vi "ReplaceSymbolValue.vi"(8 "error in (no error)":errorcluster, 11 "SetConditionalSymbol in":refnum<class "SetConditionalSymbol.lvclass">) -> (0 "error out":errorcluster, 1 "Output/Failure":string, 2 "Success?":bool, 3 "SetConditionalSymbol out":refnum<class "SetConditionalSymbol.lvclass">)   [LabVIEW 2020, in "SetConditionalSymbol.lvclass"]
doc: "Sets the value of the conditional disable symbol to what was provided to the LabVIEWCLI."
uses:
  SetConditionalSymbol.lvclass
  SetConditionalSymbol.lvclass/SetConditionalSymbol.ctl
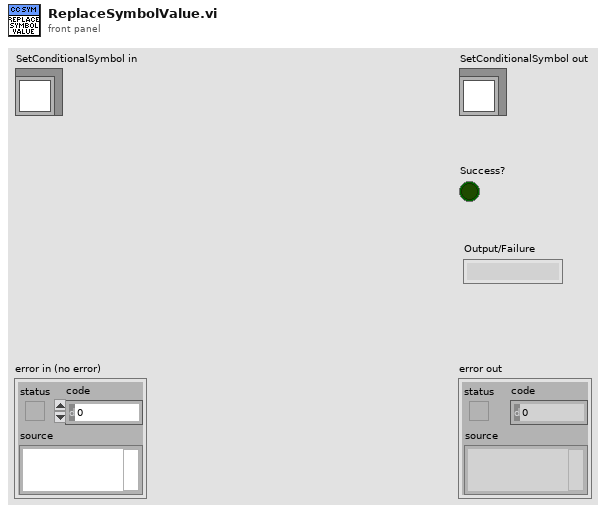
[diagram p1: front panel]
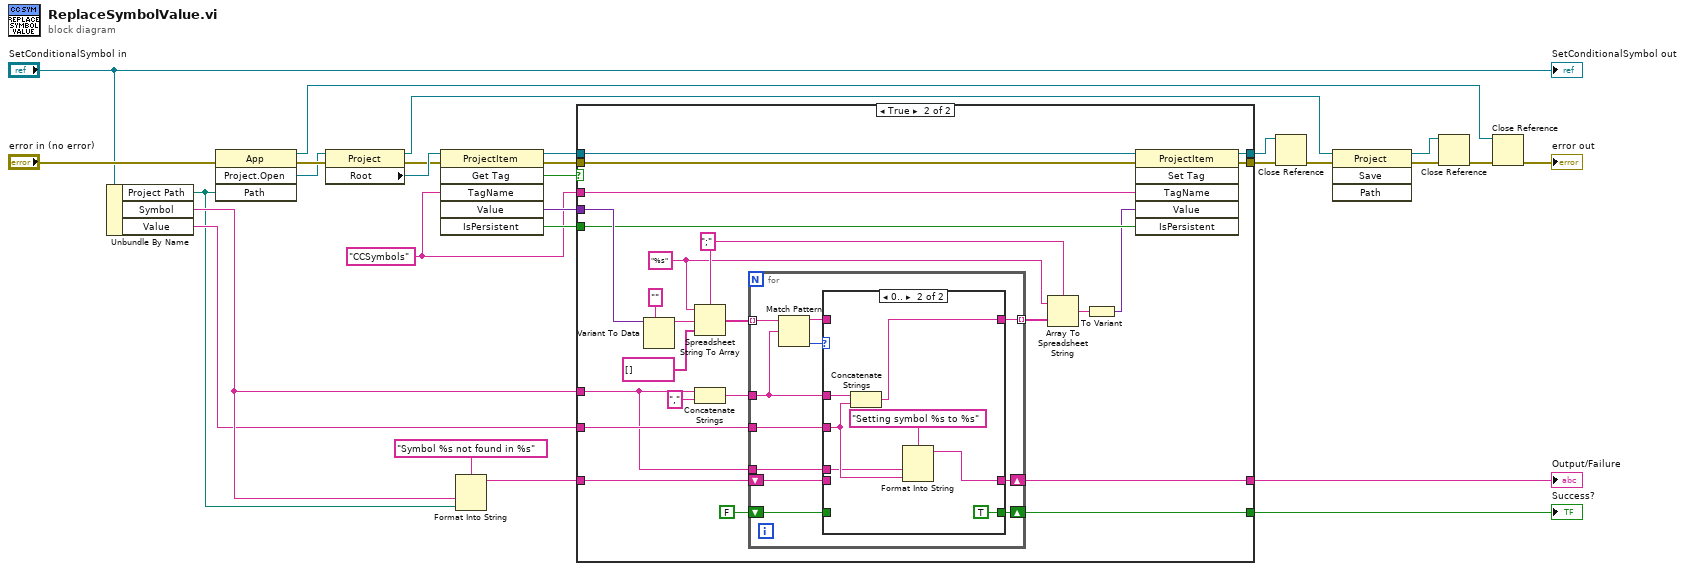
[diagram p0: block diagram]
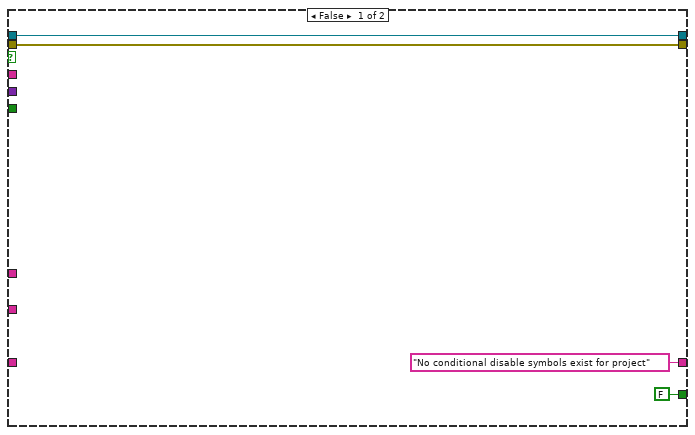
[diagram p2: hidden frame]
diagram:
  w19 = "CCSymbols" ("Tag Name")
  n1 = Unbundle By Name("SetConditionalSymbol in") -> ("Project Path"=w2:path, "Symbol"=w4:string, "Value"=w3:string)
  n2 = invoke class="App" method="Project.Open"(error in="error in (no error)", "Path"=w2) -> (reference out=w7:refnum<vi>, error out=w12:errorcluster, "Project:Open"=w11:refnum<vi>)  [unwired: 2 in, 1 out]
  n3 = property class="Project"(reference=w11, error in=w12) -> (reference out=w8:refnum<vi>, error out=w13:errorcluster, "Root"=w14:refnum<vi>)
  n4 = invoke class="ProjectItem" method="Get Tag"(reference=w14, error in=w13, "TagName"=w19) -> (reference out=w21:refnum<vi>, error out=w22:errorcluster, "GetTag"=w23:bool, "Value"=w24:variant, "IsPersistent"=w20:bool)  [unwired: 3 in, 1 out]
  n5 = Format Into String(format string="Symbol %s not found in %s" ("Tag Name"), w4, w2) -> (resulting string=w5:string)  [unwired: 2 in, 1 out]
  n6 = case shown="True" w23 {
    tunnel: w24 -> [_ w56]
    tunnel: w4 -> [_ w36]
    tunnel: w3 -> [_ w49]
    tunnel: w22 -> [w32 w44]
    tunnel: w21 -> [w31 w43]
    tunnel: [w32 w42] -> w10
    tunnel: [w31 w41] -> w9
    tunnel: w20 -> [_ w40]
    tunnel: w19 -> [_ w38]
    tunnel: w5 -> [_ w37]
    tunnel: ["No conditional disable symbols exist for project" w35] -> w25
    tunnel: [FALSE w33] -> w1
    frame False {
    }
    frame True {
      w46 = "%s" ("format string")
      w47 = ";" ("delimiter (Tab)")
      n7 = Variant To Data(type="", Variant=w56) -> (data=w54:string)  [unwired: 1 in, 1 out]
      n8 = Spreadsheet String To Array(delimiter (Tab)=w47, format string=w46, spreadsheet string=w54, array type (2D Dbl)=string[] []) -> (array=w52:string[])
      n9 = Concatenate Strings(w36, "," ("string")) -> (w50:string)
      n10 = for {
        tunnel: w52 -> [w66] mode=indexing
        tunnel: w50 -> [w62]
        tunnel: w49 -> [w63]
        tunnel: [w65] -> w48 mode=indexing
        shift-right: [w60] -> w35
        shift-left: w37 -> [w61]
        tunnel: w36 -> [w59]
        shift-right: [w57] -> w33
        shift-left: FALSE -> [w58]
        n11 = Match Pattern(string=w66, regular expression=w62) -> (before substring=w64:string, offset past match=w67:i32)  [unwired: 1 in, 2 out]
        n12 = case shown="0.." w67 {
          tunnel: w64 -> [w70 _]
          tunnel: [w70 w76] -> w65
          tunnel: w63 -> [_ w73]
          tunnel: w62 -> [_ w77]
          tunnel: w61 -> [w69 _]
          tunnel: [w69 w74] -> w60
          tunnel: w59 -> [_ w72]
          tunnel: w58 -> [w68 _]
          tunnel: [w68 TRUE] -> w57
          frame Default {
          }
          frame 0.. {
            n13 = Concatenate Strings(w77, w73) -> (w76:string)
            n14 = Format Into String(format string="Setting symbol %s to %s", w72, w73) -> (resulting string=w74:string)  [unwired: 2 in, 1 out]
          }
        }
      }
      n15 = Array To Spreadsheet String(delimiter (Tab)=w47, array=w48, 3:w46) -> (spreadsheet string=w45:string)
      n16 = To Variant(anything=w45) -> (Variant=w39:variant)
      n17 = invoke class="ProjectItem" method="Set Tag"(reference=w43, error in=w44, "TagName"=w38, "Value"=w39, "IsPersistent"=w40) -> (reference out=w41:refnum<vi>, error out=w42:errorcluster)  [unwired: 1 in, 4 out]
    }
  }
  "Output/Failure" <- w25
  "Success?" <- w1
  n18 = Close Reference(reference=w9, error in (no error)=w10) -> (error out=w18:errorcluster)
  n19 = invoke class="Project" method="Save"(reference=w8, error in=w18) -> (reference out=w16:refnum<vi>, error out=w17:errorcluster)  [unwired: 2 in, 2 out]
  n20 = Close Reference(reference=w16, error in (no error)=w17) -> (error out=w15:errorcluster)
  n21 = Close Reference(reference=w7, error in (no error)=w15) -> (error out=→"error out":errorcluster)
  "SetConditionalSymbol out" <- "SetConditionalSymbol in"
